vi "TDT-Get Events (Tosca).vi"(0 "Data":T1={"TTankX"=refnum, "TDevAccX"=refnum, "LastTime"=0.0, "error"={"status"=FALSE, "code"=0, "source"=""}, "Block Name"="", "Circuit Tag"="", "Tank Name"="", "NumTicks"=0, "LastTick"=0.0, "Idle?"=FALSE, "Wait (ms)"=1000, "LastArtf"=0.0, "LastTosc"=0.0}, 7 "Max Read":i32=20000, 11 "error in (no error)":errorcluster, 13 "Tetrode":bool) -> (4 "Data out":T1={"TTankX"=refnum, "TDevAccX"=refnum, "LastTime"=0.0, "error"={"status"=FALSE, "code"=0, "source"=""}, "Block Name"="", "Circuit Tag"="", "Tank Name"="", "NumTicks"=0, "LastTick"=0.0, "Idle?"=FALSE, "Wait (ms)"=1000, "LastArtf"=0.0, "LastTosc"=0.0}, 8 "Events":dbl[][](array[numeric]), 15 "error out":errorcluster)   [LabVIEW 2015]
uses:
  TDT Interface Data.ctl
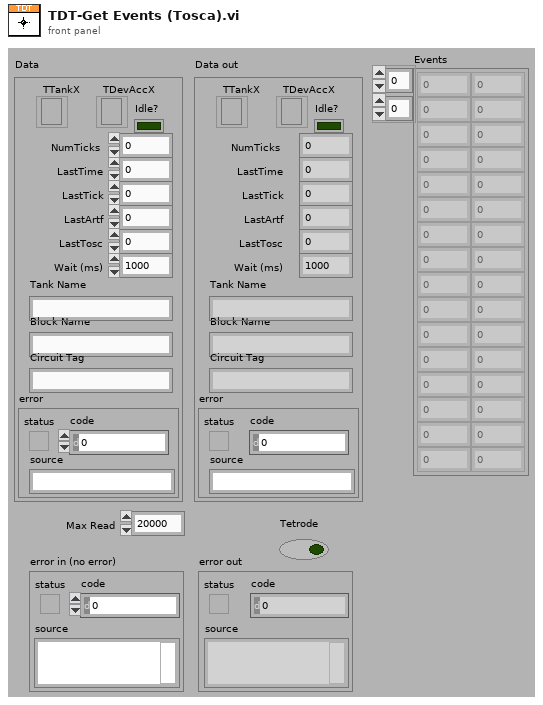
[diagram p1: front panel]
types:
  T1 = typedef "TDT Interface Data.ctl" = cluster{"TTankX":refnum<k7>, "TDevAccX":refnum<k7>, "LastTime":dbl, "error":errorcluster, "Block Name":string, "Circuit Tag":string, "Tank Name":string, "NumTicks":i32, "LastTick":dbl, "Idle?":bool, "Wait (ms)":u32, "LastArtf":dbl, "LastTosc":dbl}
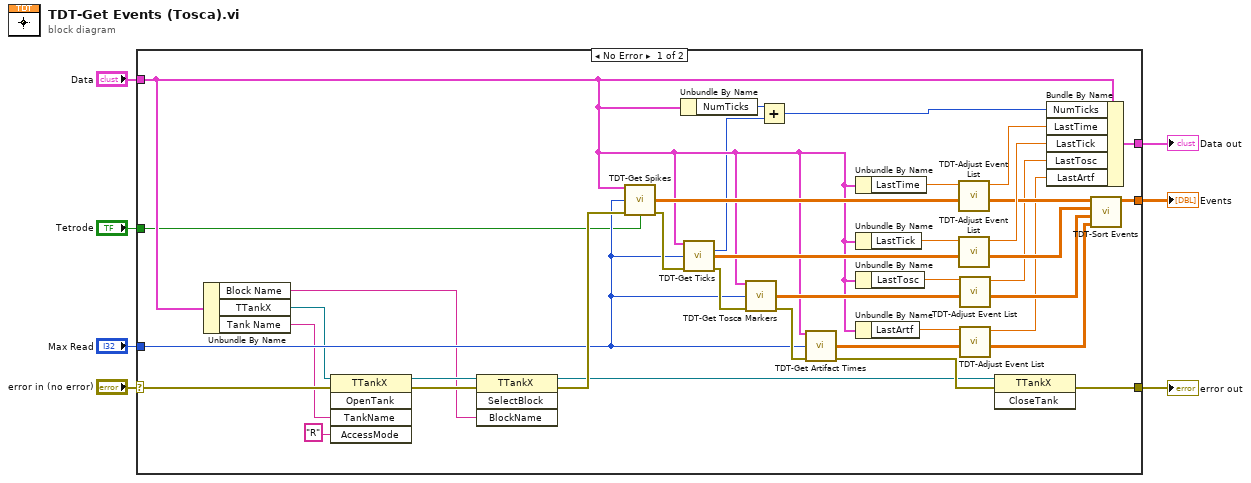
[diagram p0: block diagram]
diagram:
  n1 = case shown="No Error" "error in (no error)" {
    selector: "error in (no error)" -> [w20 w47]
    tunnel: [w19 w47] -> w6
    tunnel: "Data" -> [w12 w46]
    tunnel: "Max Read" -> [w21 _]
    tunnel: [w35 _] -> w3
    tunnel: [w43 w46] -> w2
    tunnel: "Tetrode" -> [w8 _]
    frame No Error {
      n2 = Unbundle By Name(w12) -> ("Block Name"=w14:string, "TTankX"=w10:refnum<k7>, "Tank Name"=w15:string)
      n3 = invoke class="TTankX" method="OpenTank"(reference=w10, error in=w20, "TankName"=w15, "AccessMode"="R") -> (reference out=w16:refnum<k7>, error out=w17:errorcluster)  [unwired: 1 in, 3 out]
      n4 = invoke class="TTankX" method="SelectBlock"(reference=w16, error in=w17, "BlockName"=w14) -> (reference out=w11:refnum<k7>, error out=w32:errorcluster)  [unwired: 1 in, 2 out]
      n5 = call "TDT-Get Spikes.vi"("Data"=w12, "Max Read"=w21, "error in (no error)"=w32, "Tetrode"=w8) -> ("Spike times"=w39:dbl[][], "error out"=w45:errorcluster)  [unwired: 8 in, 2 out]
      n6 = Unbundle By Name(w12) -> ("NumTicks"=w44:i32)
      n7 = call "TDT-Get Ticks.vi"("Data"=w12, "Max Read"=w21, "error in (no error)"=w45) -> ("Number of Ticks"=w9:i32, "Tick times"=w38:dbl[][], "error out"=w31:errorcluster)  [unwired: 9 in, 1 out]
      n8 = call "TDT-Get Tosca Markers.vi"("Data"=w12, "Max Read"=w21, "error in (no error)"=w31) -> ("Tosca markers"=w30:dbl[][], "error out"=w22:errorcluster)  [unwired: 10 in, 1 out]
      n9 = Add(x=w44, y=w9) -> (x+y=w42:i32)
      n10 = call "TDT-Get Artifact Times.vi"("Data"=w12, "Max Read"=w21, "error in (no error)"=w22) -> ("Artifact Times"=w23:dbl[][], "error out"=w18:errorcluster)  [unwired: 10 in, 1 out]
      n11 = Unbundle By Name(w12) -> ("LastTime"=w41:dbl)
      n12 = Unbundle By Name(w12) -> ("LastTick"=w37:dbl)
      n13 = Unbundle By Name(w12) -> ("LastTosc"=w29:dbl)
      n14 = Unbundle By Name(w12) -> ("LastArtf"=w24:dbl)
      n15 = call "TDT-Adjust Event List.vi"("Events in"=w39, "Last In"=w41) -> ("Events out"=w34:dbl[][], "Last out"=w40:dbl)  [unwired: 8 in]
      n16 = call "TDT-Adjust Event List.vi"("Events in"=w38, "Last In"=w37) -> ("Events out"=w33:dbl[][], "Last out"=w36:dbl)  [unwired: 8 in]
      n17 = call "TDT-Adjust Event List.vi"("Events in"=w30, "Last In"=w29) -> ("Events out"=w27:dbl[][], "Last out"=w28:dbl)  [unwired: 8 in]
      n18 = call "TDT-Adjust Event List.vi"("Events in"=w23, "Last In"=w24) -> ("Events out"=w26:dbl[][], "Last out"=w25:dbl)  [unwired: 8 in]
      n19 = invoke class="TTankX" method="CloseTank"(reference=w11, error in=w18) -> (error out=w19:errorcluster)  [unwired: 1 in, 2 out]
      n20 = Bundle By Name(cluster=w12, "NumTicks"=w42, "LastTime"=w40, "LastTick"=w36, "LastTosc"=w28, "LastArtf"=w25) -> (w43:T1)
      n21 = call "TDT-Sort Events.vi"("Tosca Markers"=w26, "Artifacts"=w27, "Spikes"=w33, "Ticks"=w34) -> ("Sorted events"=w35:dbl[][])  [unwired: 7 in]
    }
    frame Error {
    }
  }
  "error out" <- w6
  "Data out" <- w2
  "Events" <- w3
